vi "Read Data.vi"() -> ()   [LabVIEW 2014]
panel:
  out "Data Chart":dbl(graph)
  in  "stop":bool
  in  "Time Delay (ms)":dbl(slide) scale=0.0..10.0
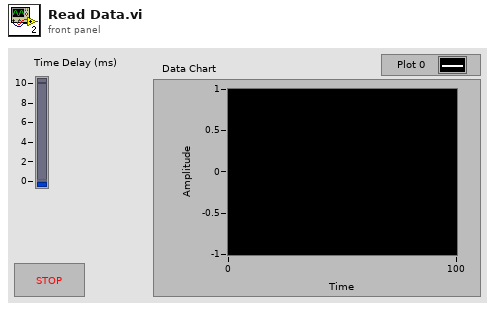
[diagram p1: front panel]
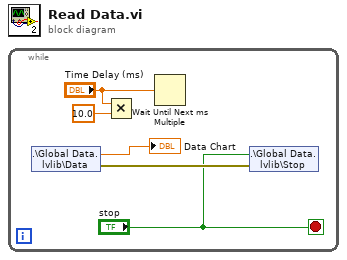
[diagram p0: block diagram]
diagram:
  n1 = while {
    stop <- "stop" stop-if-true
    n2 = shared-variable ".\\Global Data.lvlib\\Data"() -> (→"Data Chart":dbl, error out=w4:errorcluster)  [unwired: 1 in]
    n3 = Multiply(x="Time Delay (ms)", y=10.0) -> ()  [unwired: 1 out]
    n4 = Wait Until Next ms Multiple(millisecond multiple="Time Delay (ms)") -> ()  [unwired: 1 out]
    n5 = shared-variable ".\\Global Data.lvlib\\Stop"("stop", error in=w4) -> ()  [unwired: 1 out]
  }
